vi "Digital Burst Named Pattern.vi"(7 "Pattern Names":string[](array[string]), 10 "Pin Names":string[](array[string]), 11 "Semiconductor Module Context":T1) -> (0 "error out":errorcluster, 3 "pass":bool[](array[boolean]))   [LabVIEW 2014]
uses:
  <vilib>/NI_TestStand_SemiconductorModule/NI_TestStand_Semiconductor_Module.lvlibp/PinMap/General/SemiconductorModuleContext.ctl
  <vilib>/NI_TestStand_SemiconductorModule/NI_TestStand_Semiconductor_Module.lvlibp/PinMap/Digital Pattern/PinsToNIDigitalPatternSessions.vi
  <instrlib>/niDigital/niDigital.llb/niDigital Burst Pattern (Pass Fail).vi
  <vilib>/NI_TestStand_SemiconductorModule/NI_TestStand_Semiconductor_Module.lvlibp
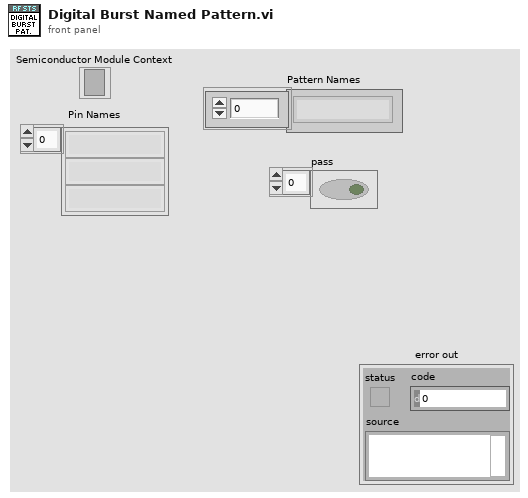
[diagram p1: front panel]
types:
  T1 = typedef "NI_TestStand_Semiconductor_Module.lvlibp/SemiconductorModuleContext.ctl" = refnum<k7>
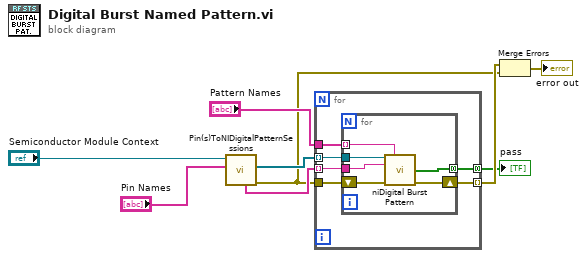
[diagram p0: block diagram]
diagram:
  n1 = call-poly <vilib>:"Pin(s)ToNIDigitalPatternSessions.vi"("Pins"="Pin Names", "Semiconductor Module Context"="Semiconductor Module Context") -> ("error out"=w2:errorcluster, "Instrument Sessions"=w7:refnum<k15>[], "Site Lists"=w5:string[])  [unwired: 4 in, 3 out]
  n2 = for {
    tunnel: w7 -> [w12] mode=indexing
    tunnel: "Pattern Names" -> [w15]
    tunnel: w5 -> [w13] mode=indexing
    tunnel: w2 -> [w11]
    tunnel: [w14] -> w3 mode=indexing
    tunnel: [w10] -> w1 mode=concatenating
    n3 = for {
      tunnel: w15 -> [w21] mode=indexing
      tunnel: w12 -> [w18]
      shift-right: [w20] -> w14
      shift-left: w11 -> [w19]
      tunnel: w13 -> [w17]
      tunnel: [w16] -> w10 mode=concatenating
      n4 = call-poly <instrlib>:"niDigital Burst Pattern.vi"("instrument handle"=w18, "start label"=w21, "site list"=w17, "error in"=w19) -> ("pass"=w16:bool[], "error out"=w20:errorcluster)  [unwired: 9 in, 1 out]
    }
  }
  "pass" <- w1
  n5 = Merge Errors(w3, w2) -> (→"error out":errorcluster)
